vi "NavX Close.vi"(8 "error in":errorcluster) -> (0 "error out":errorcluster)   [LabVIEW 2014]
uses:
  Global Objects.vi
  navX Library v2/navX Library v2.lvlib
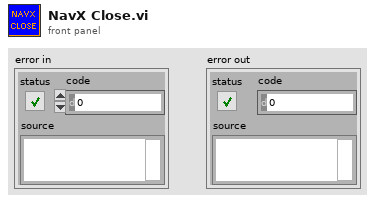
[diagram p1: front panel]
types:
  T1 = typedef "NaxX Info.ctl" = cluster{"navX Device":T2, "Previous Heading":dbl}
  T2 = typedef "navX Library v2.lvlib/Z900_navX_DeviceTypeDef.ctl" = cluster{"Interface":cluster{"Protocol":T3, "Update Rate (4Hz-60Hz)":u8, "navX Open TypeDef":variant}, "Notify Packet":refnum<notifier>, "Loop VI Refnum":refnum<vi>, "Ready to Close Occurrence Refnum":refnum<k4>}
  T3 = typedef "navX Library v2.lvlib/Z900_navX_ProtocolTypeDef.ctl" = enum16{"SERIAL", "I2C", "SPI"}
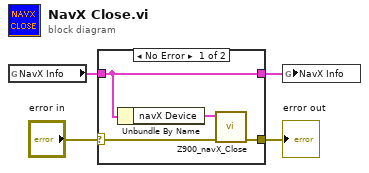
[diagram p0: block diagram]
diagram:
  n1 = global read "Global Objects.vi" "NavX Info"() -> (w2:T1)
  n2 = case shown="No Error" "error in" {
    selector: "error in" -> [w7 w10]
    tunnel: [w6 w10] -> w3
    tunnel: w2 -> [w5 w9]
    tunnel: [w5 w9] -> w1
    frame No Error {
      n3 = Unbundle By Name(w5) -> ("navX Device"=w8:T2)
      n4 = call "Z900_navX_Close.vi"("error in (no error)"=w7, "navX Device"=w8) -> ("error out"=w6:errorcluster)  [unwired: 9 in]
    }
    frame Error {
    }
  }
  "error out" <- w3
  n5 = global write "Global Objects.vi" "NavX Info"(w1) -> ()
